vi "basic signals using case structure.vi"() -> ()   [LabVIEW 2020]
uses:
  <vilib>/measure/NI_MABase.lvlib
panel:
  in  "stop":bool
  in  "signal type":T1(ring)
  out "Waveform Graph":waveform(dbl)(graph)
  in  "amplitude":dbl(knob) scale=0.0..10.0
  in  "frequency":dbl(knob) scale=0.0..10.0
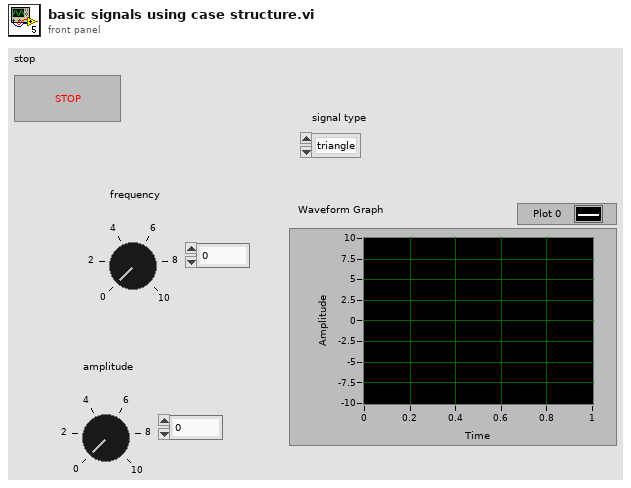
[diagram p1: front panel]
types:
  T1 = enum16{"triangle", "saw tooth", "square", "sine"}
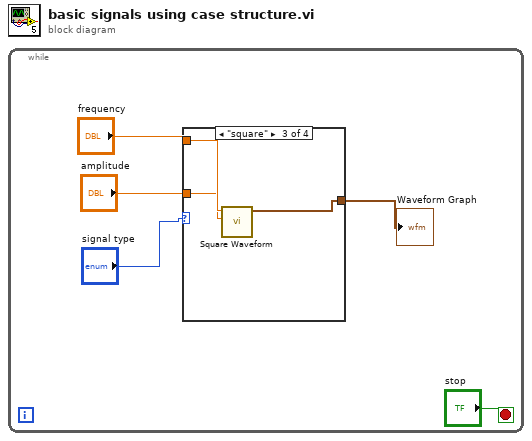
[diagram p0: block diagram]
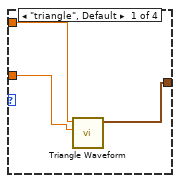
[diagram p2: hidden frame]
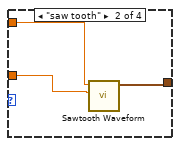
[diagram p3: hidden frame]
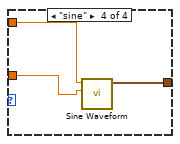
[diagram p4: hidden frame]
diagram:
  n1 = while {
    stop <- "stop" stop-if-true
    n2 = case shown="\"square\"" "signal type" {
      tunnel: "frequency" -> [w8 w11 w14 w17]
      tunnel: "amplitude" -> [w7 w10 w13 w16]
      tunnel: [w6 w9 w12 w15] -> w1
      frame "triangle", Default {
        n3 = call <vilib>:"Triangle Waveform.vi"("amplitude"=w7, "frequency"=w8) -> ("signal out"=w6:waveform(dbl))  [unwired: 8 in, 1 out]
      }
      frame "saw tooth" {
        n4 = call <vilib>:"Sawtooth Waveform.vi"("amplitude"=w10, "frequency"=w11) -> ("signal out"=w9:waveform(dbl))  [unwired: 8 in, 1 out]
      }
      frame "square" {
        n5 = call <vilib>:"Square Waveform.vi"("amplitude"=w13, "frequency"=w14) -> ("signal out"=w12:waveform(dbl))  [unwired: 8 in, 1 out]
      }
      frame "sine" {
        n6 = call <vilib>:"Sine Waveform.vi"("amplitude"=w16, "frequency"=w17) -> ("signal out"=w15:waveform(dbl))  [unwired: 8 in, 1 out]
      }
    }
    "Waveform Graph" <- w1
  }
